vi "Display.vi"(8 "error in (no error)":errorcluster, 10 "SubPnl":refnum<vi>, 11 "Configurator Base in":refnum<class "Configurator Base.lvclass">) -> (0 "error out":errorcluster, 3 "Configurator Base out":refnum<class "Configurator Base.lvclass">)   [LabVIEW 2023, in "Configurator Base.lvclass"]
uses:
  Configurator Base.lvclass
  Configurator Base.lvclass/Configurator Base.ctl
panel:
  in  "Instr Configuration":string
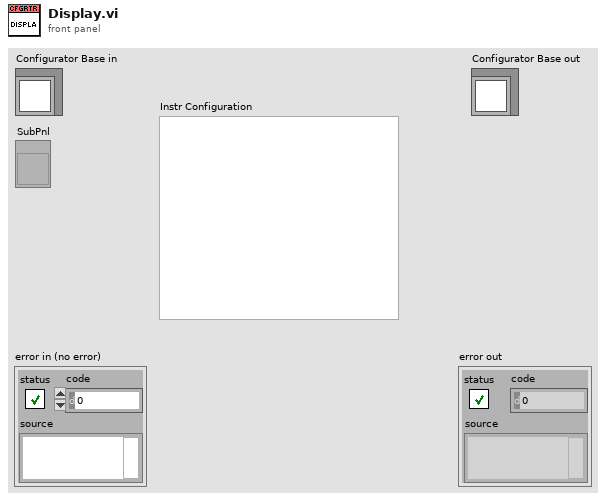
[diagram p1: front panel]
types:
  T1 = enum32{"Invalid", "Standard", "Closed", "Hidden", "Minimized", "Maximized"}
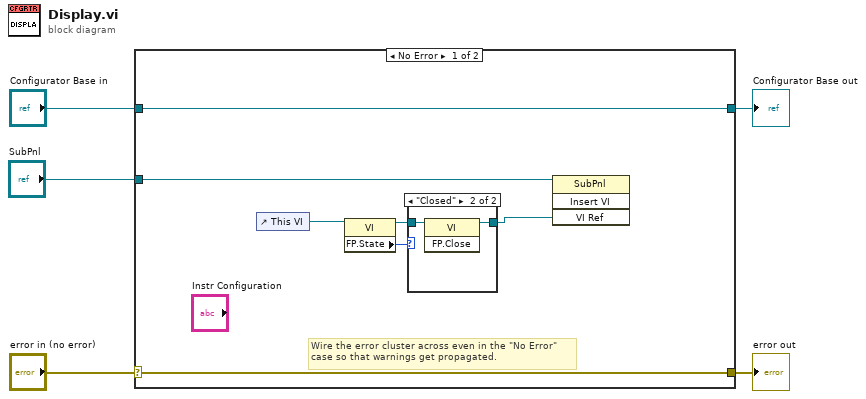
[diagram p0: block diagram]
diagram:
  n1 = case shown="No Error" "error in (no error)" {
    selector: "error in (no error)" -> [w11 w16]
    tunnel: [w11 w16] -> w4
    tunnel: [w12 w15] -> w2
    tunnel: "Configurator Base in" -> [w12 w15]
    tunnel: "SubPnl" -> [w7 _]
    frame No Error {
      # "Wire the error cluster across even in the \"No Error\"\ncase so that warnings get propagated."
      n2 = control-ref of="This VI"() -> (w10:refnum<vi>)
      n3 = property class="VI"(reference=w10) -> (reference out=w8:refnum<vi>, "FP.State"=w9:T1)  [unwired: 1 in, 1 out]
      n4 = case shown="\"Closed\"" w9 {
        tunnel: w8 -> [_ w14]
        tunnel: [_ w13] -> w6
        frame Default {
        }
        frame "Closed" {
          n5 = invoke class="VI" method="FP.Close"(reference=w14) -> (reference out=w13:refnum<vi>)  [unwired: 2 in, 2 out]
        }
      }
      n6 = invoke class="SubPnl" method="Insert VI"(reference=w7, "VI Ref"=w6) -> ()  [unwired: 2 in, 4 out]
    }
    frame Error {
    }
  }
  "error out" <- w4
  "Configurator Base out" <- w2
